vi "3.手柄操作发送指令至TCP服务器.vi"() -> ()   [LabVIEW 2018]
uses:
  <vilib>/Utility/inputDevices.llb/joystickAcquire.vi
panel:
  in  "摄像头云台复位":bool
  in  "运动控制复位":bool
  in  "摄像头云台负向1":bool
  in  "摄像头云台正向1":bool
  in  "摄像头正向2":bool
  in  "摄像头负向2":bool
  in  "机械手扩展":bool
  in  "机械手夹紧":bool
  in  "重新采样":bool
  in  "水下采样":bool
  in  "右旋":bool
  in  "左旋":bool
  in  "右翻":bool
  in  "左翻":bool
  in  "下潜":bool
  in  "上浮":bool
  in  "后退":bool
  in  "右移":bool
  in  "左移":bool
  in  "前进":bool
  out "接收字符串":string
  out "开始flag":bool=TRUE
  in  "?":string="8088"
  in  "?":string="192.168.1.30"
  # "地   址："
  # "端口号："
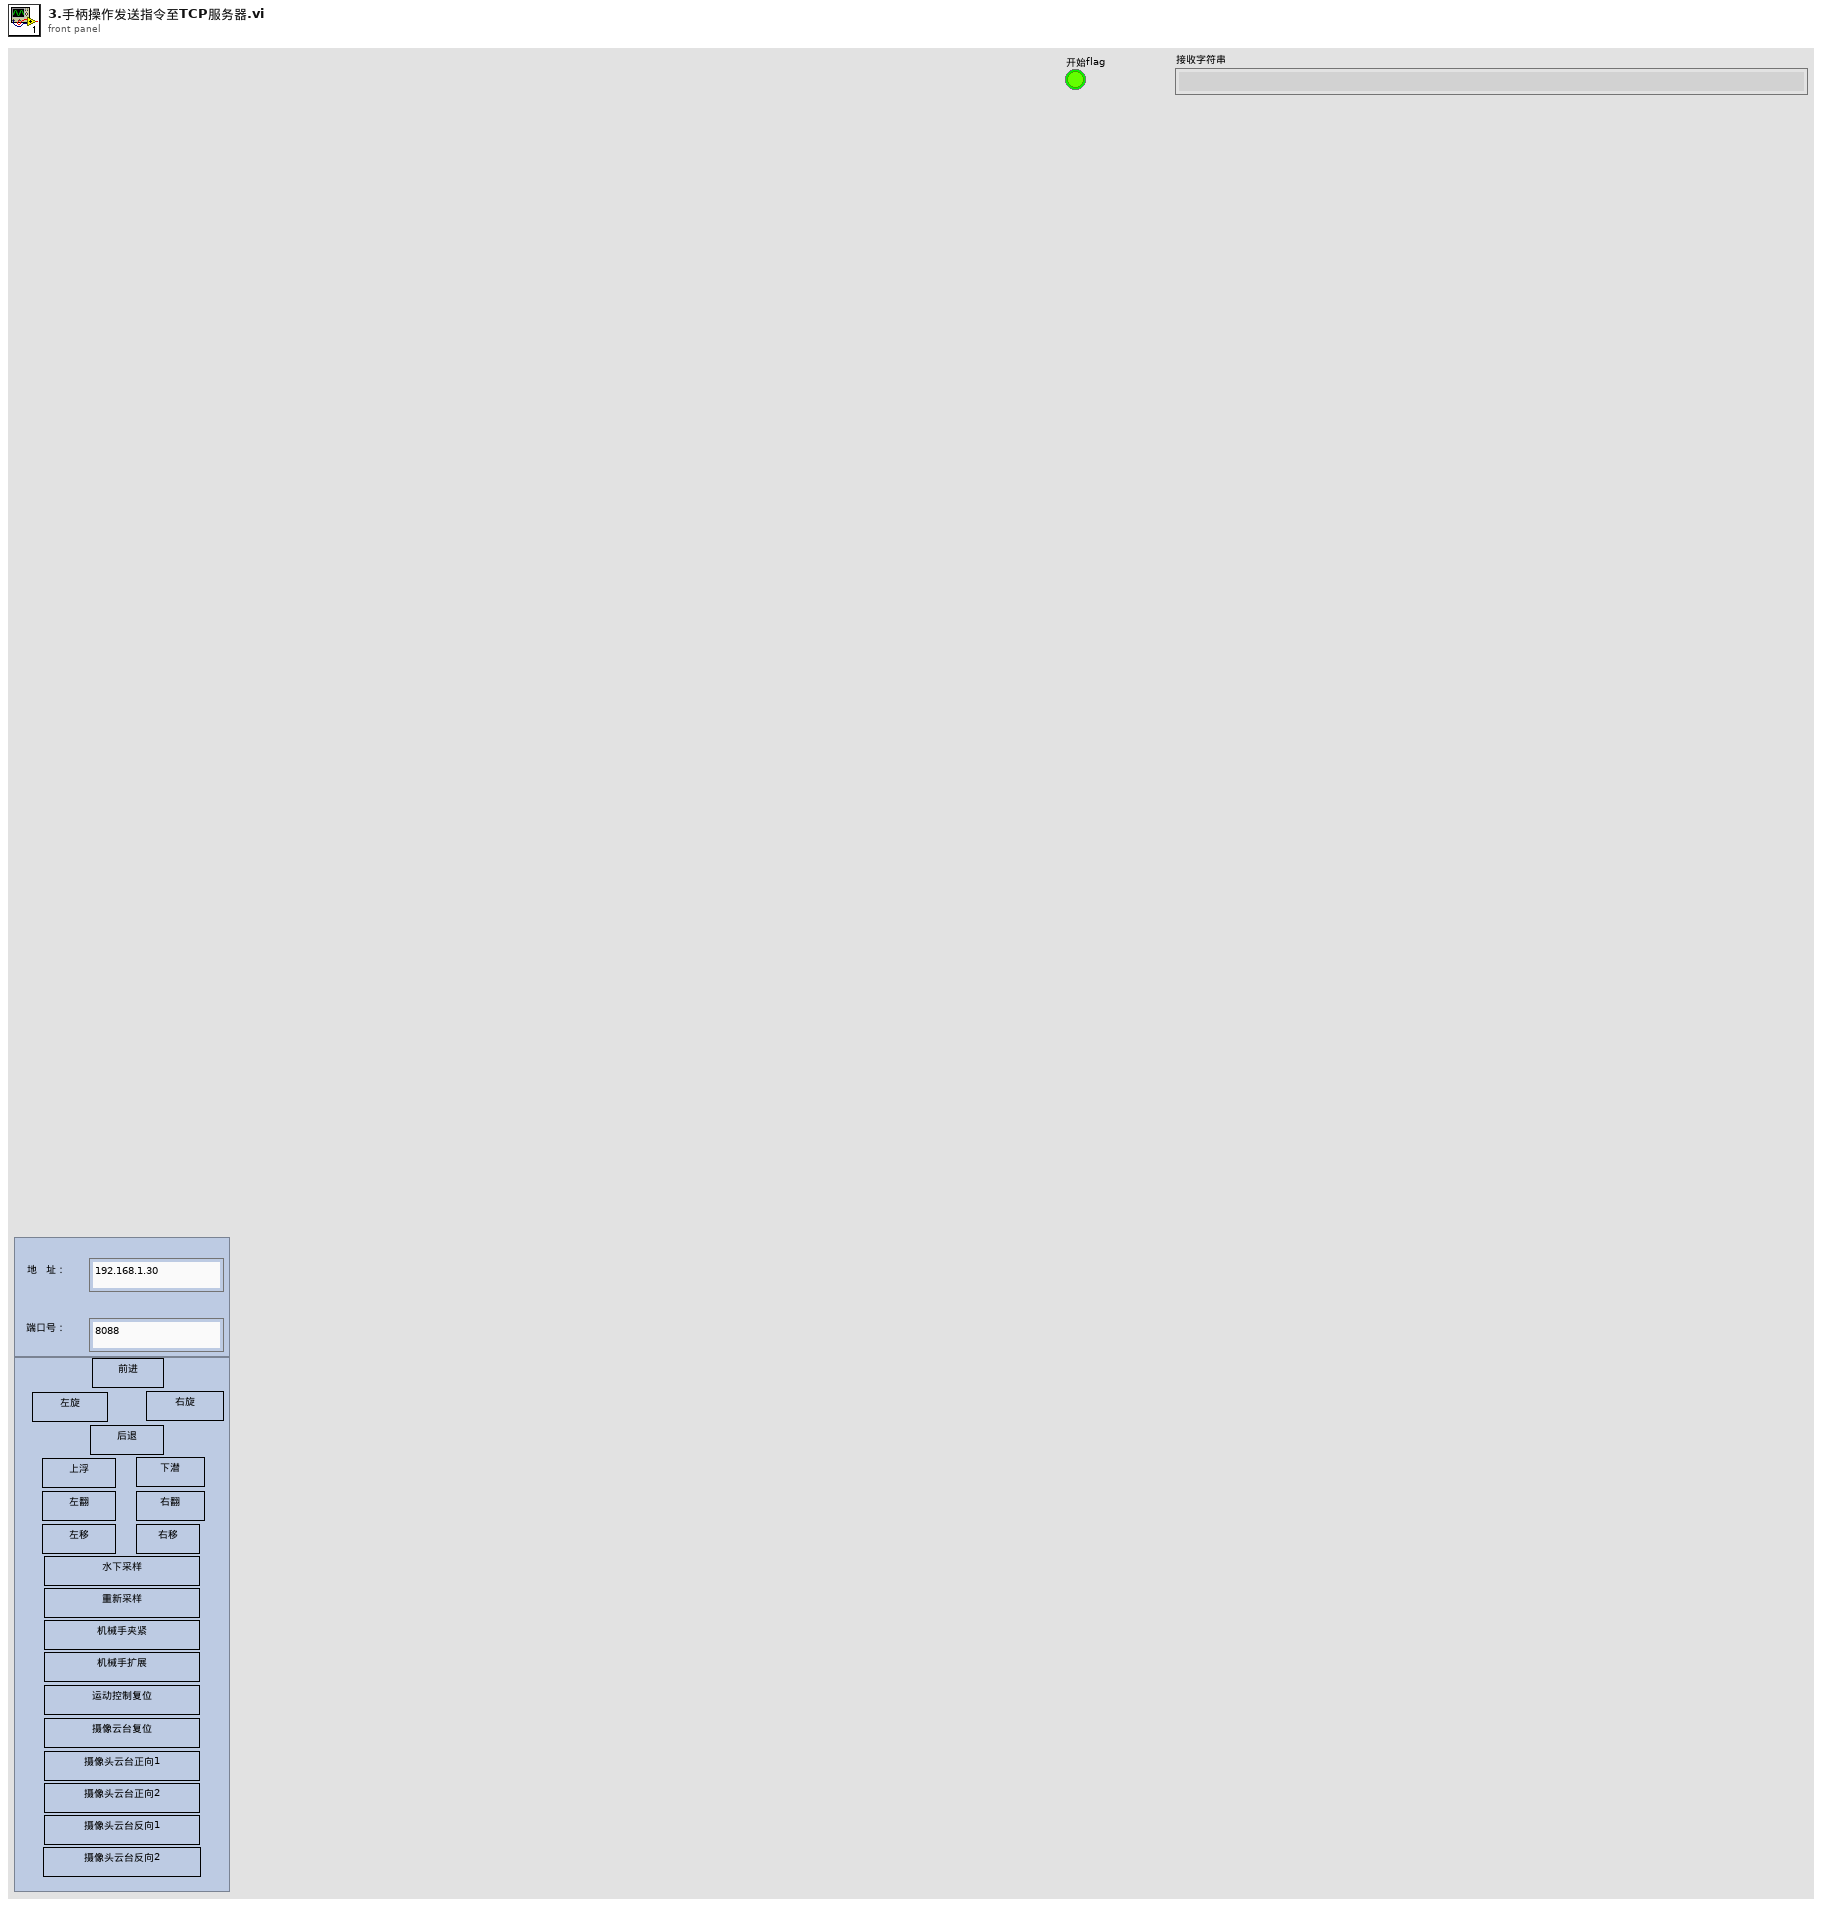
[diagram p1: front panel]
types:
  T1 = cluster{"X axis":i32, "Y axis":i32, "Z axis":i32, "X axis rotation":i32, "Y axis rotation":i32, "Z axis rotation":i32, "U axis":i32, "V axis":i32}
  T2 = cluster{"button 1":bool, "button 2":bool, "button 3":bool, "button 4":bool, "button 5":bool, "button 6":bool, "button 7":bool, "button 8":bool, "button 9":bool, "button 10":bool, "button 11":bool, "button 12":bool, "button 13":bool, "button 14":bool, "button 15":bool, "button 16":bool, "button 17":bool, "button 18":bool, "button 19":bool, "button 20":bool, "button 21":bool, "button 22":bool, "button 23":bool, "button 24":bool, "button 25":bool, "button 26":bool, "button 27":bool, "button 28":bool, "button 29":bool, "button 30":bool, "button 31":bool, "button 32":bool}
  T3 = cluster{"pov 1":i32, "pov 2":i32, "pov 3":i32, "pov 4":i32}
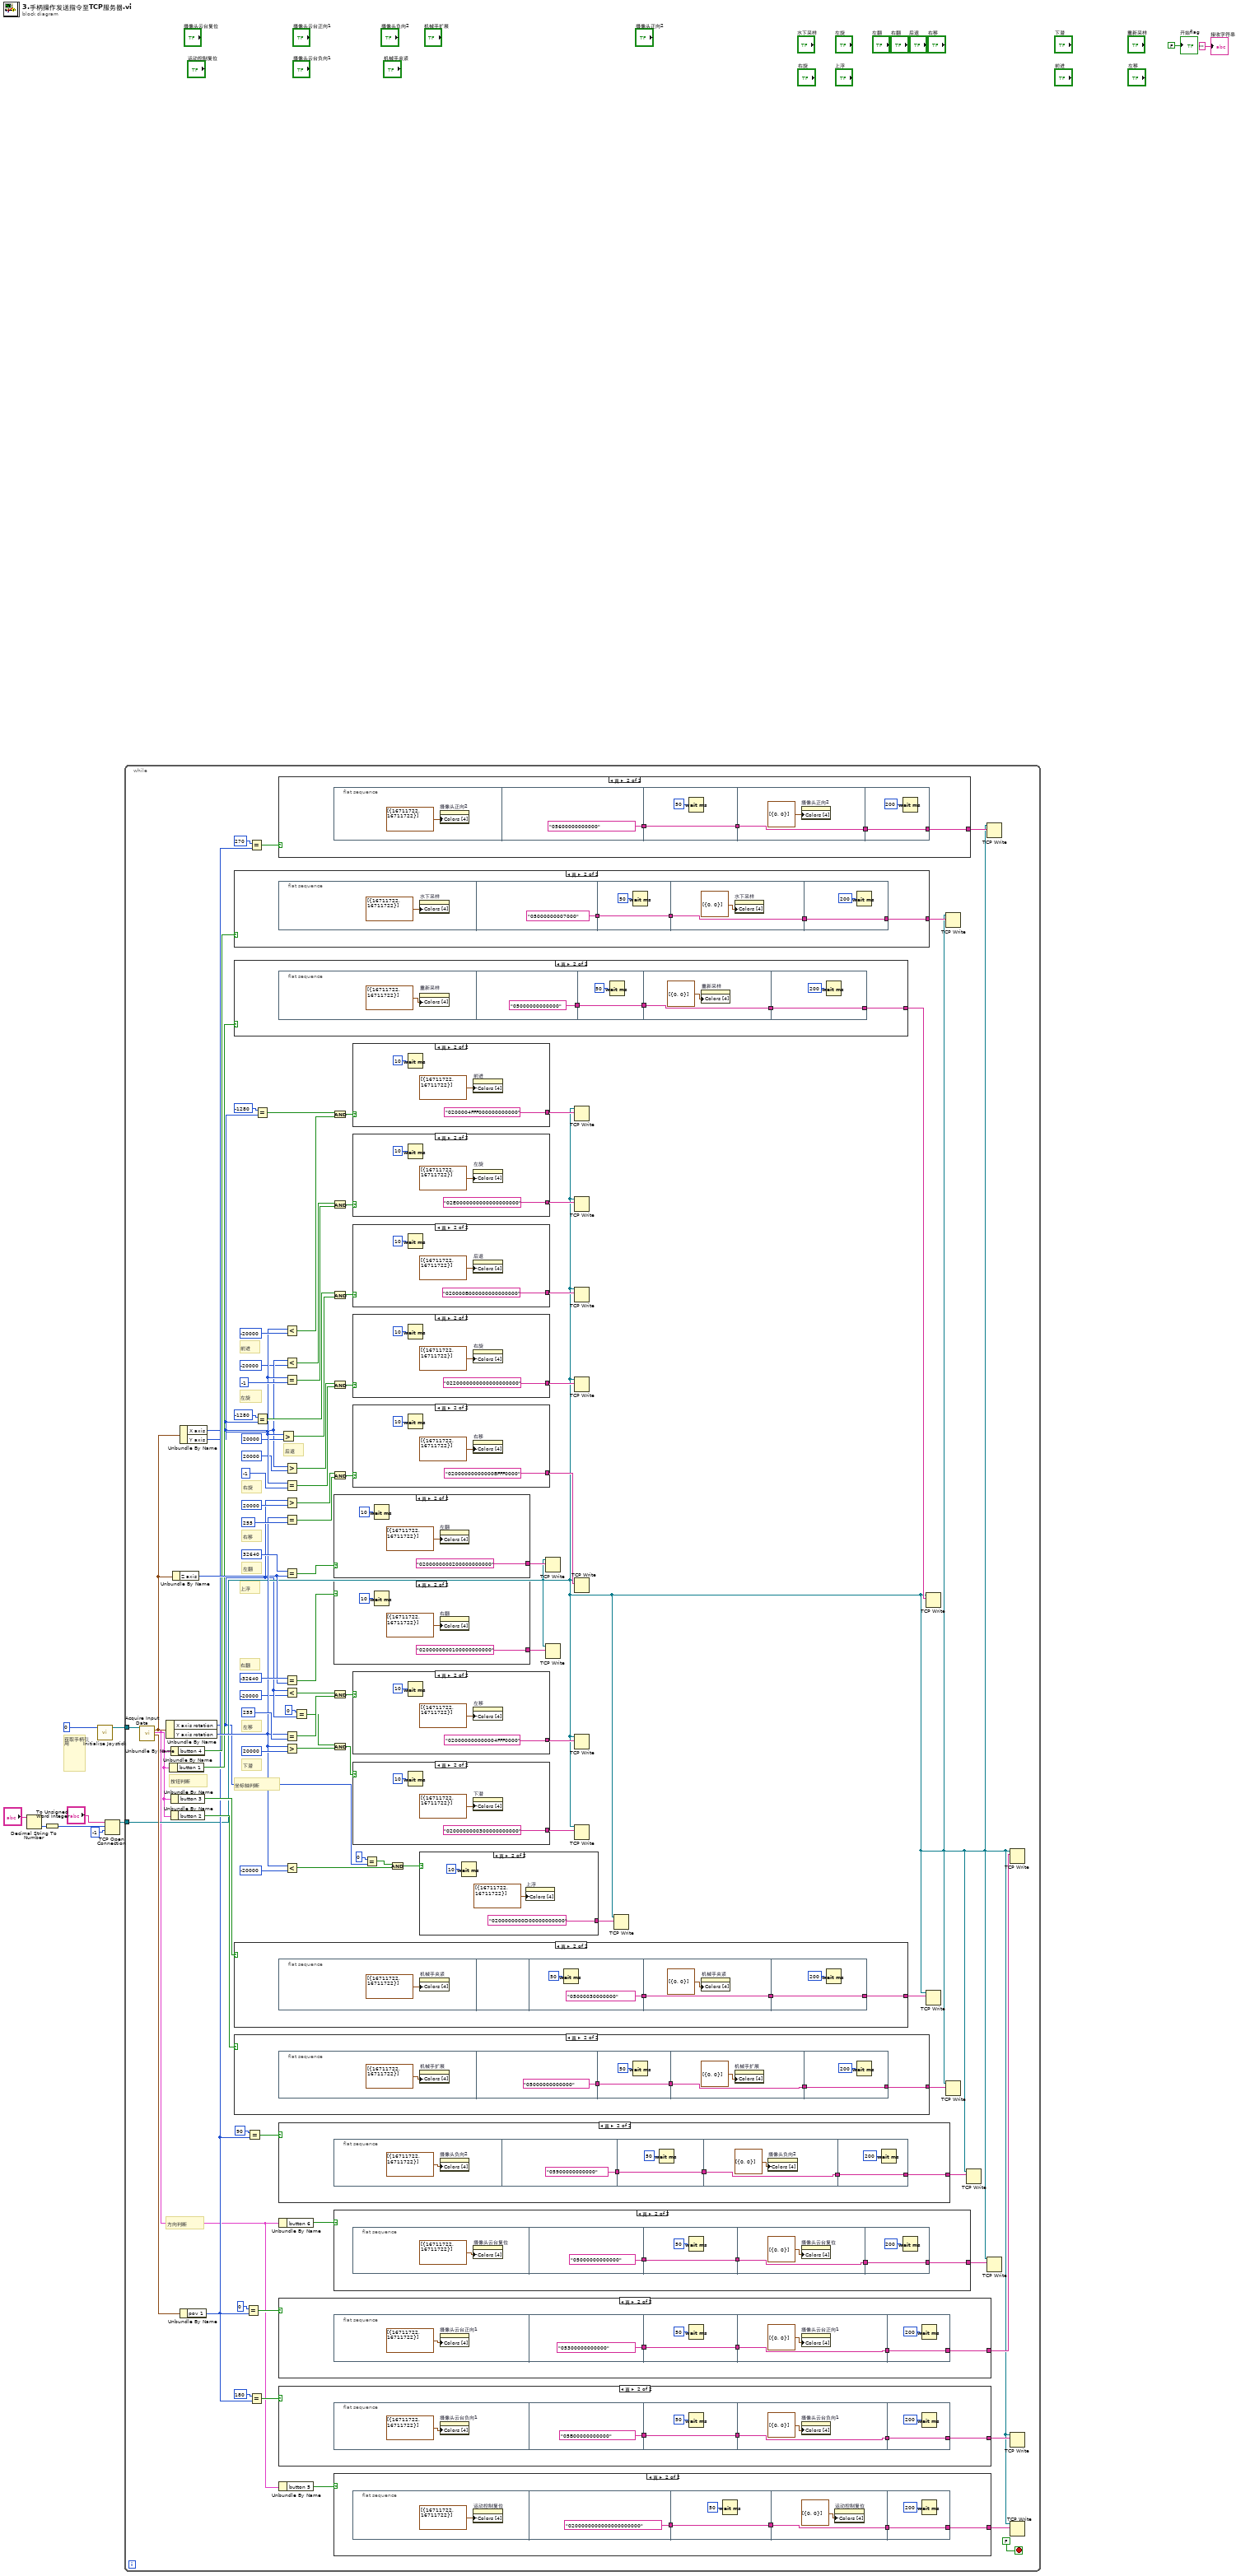
[diagram p0: block diagram]
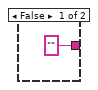
[diagram p2: hidden frame]
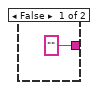
[diagram p3: hidden frame]
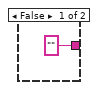
[diagram p4: hidden frame]
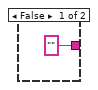
[diagram p5: hidden frame]
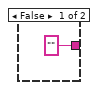
[diagram p6: hidden frame]
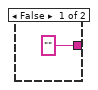
[diagram p7: hidden frame]
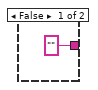
[diagram p8: hidden frame]
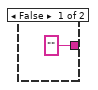
[diagram p9: hidden frame]
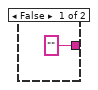
[diagram p10: hidden frame]
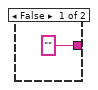
[diagram p11: hidden frame]
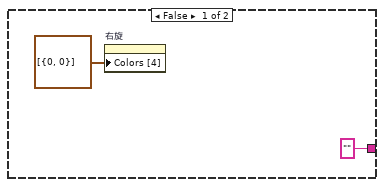
[diagram p12: hidden frame]
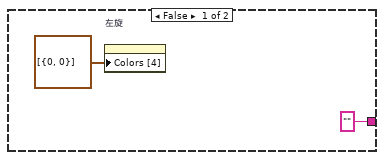
[diagram p13: hidden frame]
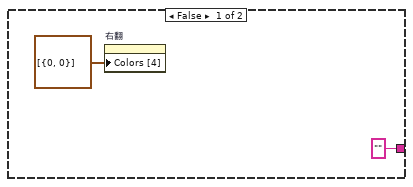
[diagram p14: hidden frame]
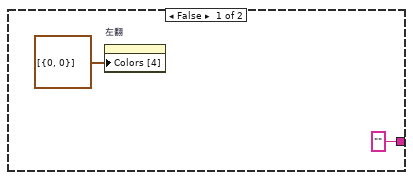
[diagram p15: hidden frame]
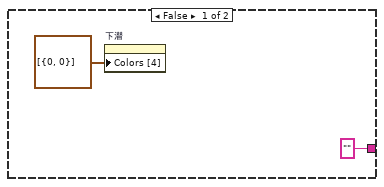
[diagram p16: hidden frame]
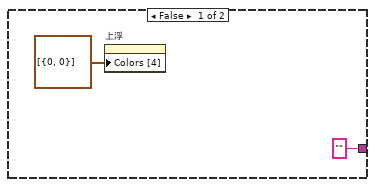
[diagram p17: hidden frame]
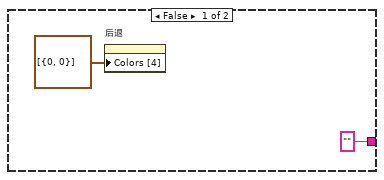
[diagram p18: hidden frame]
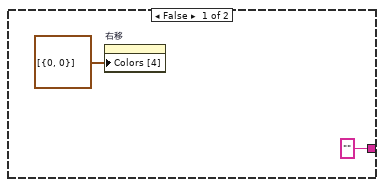
[diagram p19: hidden frame]
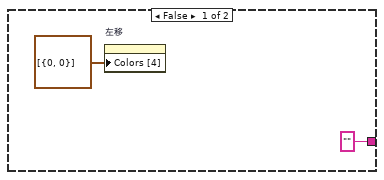
[diagram p20: hidden frame]
diagram:
  # "获取手柄引用"
  n1 = Decimal String To Number(string="?") -> (number=w6:i32)  [unwired: 2 in, 1 out]
  n2 = To Unsigned Word Integer(number=w6) -> (unsigned 16bit integer=w5:u16)
  n3 = call <vilib>:"Initialize Joystick.vi"("device index"=0) -> ("device ID"=w1:refnum<k1>)  [unwired: 9 in, 1 out]
  n4 = TCP Open Connection(address="?", remote port or service name=w5, timeout ms (60000)=-1 ("超时毫秒(60000)")) -> (connection ID=w4:refnum<k5>)  [unwired: 2 in, 1 out]
  n5 = while {
    tunnel: w4 -> [w31]
    tunnel: w1 -> [w12]
    stop <- FALSE stop-if-true
    # "方向判断"
    # "按钮判断"
    # "坐标轴判断"
    # "左翻"
    # "右旋"
    # "左旋"
    # "右翻"
    # "下潜"
    # "上浮"
    # "后退"
    # "右移"
    # "左移"
    # "前进"
    n6 = call-poly <vilib>:"Acquire Input Data.vi"("device ID"=w12) -> ("axis info"=w65:T1, "button info"=w13:T2, "direction info"=w60:T3)  [unwired: 14 in, 2 out]
    n7 = Unbundle By Name(w65) -> ("X axis rotation"=w15:i32, "Y axis rotation"=w69:i32)
    n8 = Unbundle By Name(w13) -> ("button 1"=w63:bool)
    n9 = Unbundle By Name(w13) -> ("button 4"=w64:bool)
    n10 = Unbundle By Name(w13) -> ("button 3"=w62:bool)
    n11 = Unbundle By Name(w13) -> ("button 2"=w61:bool)
    n12 = Unbundle By Name(w65) -> ("Z axis"=w66:i32)
    n13 = Unbundle By Name(w65) -> ("X axis"=w18:i32, "Y axis"=w23:i32)
    n14 = Unbundle By Name(w60) -> ("pov 1"=w56:i32)
    n15 = case shown="真" w64 {
      tunnel: ["" w217] -> w40
      frame False {
      }
      frame True {
        n16 = flat-sequence {
          tunnel: ["05000000007000"] -> w220
          tunnel: w220 -> [w223]
          tunnel: [w223] -> w219
          tunnel: w219 -> [w225]
          tunnel: [w225] -> w218
          tunnel: w218 -> [w227]
          tunnel: [w227] -> w217
          frame #0 {
            n17 = property on="水下采样" class="Bool"("Colors [4]"=cluster{u32, u32}[] [{16711722, 16711722}] ("颜色[4]")) -> ()  [unwired: 2 in, 2 out]
          }
          frame #1 {
          }
          frame #2 {
            n18 = Wait (ms)(milliseconds to wait=u32 50 ("等待时间（毫秒）")) -> ()  [unwired: 1 out]
          }
          frame #3 {
            n19 = property on="水下采样" class="Bool"("Colors [4]"=cluster{u32, u32}[] [{0, 0}] ("颜色[4]")) -> ()  [unwired: 2 in, 2 out]
          }
          frame #4 {
            n20 = Wait (ms)(milliseconds to wait=u32 200 ("等待时间（毫秒）")) -> ()  [unwired: 1 out]
          }
        }
      }
    }
    n21 = case shown="真" w63 {
      tunnel: ["" w193] -> w41
      frame False {
      }
      frame True {
        n22 = flat-sequence {
          tunnel: ["05000000000000"] -> w191
          tunnel: [w197] -> w194
          tunnel: w191 -> [w197]
          tunnel: w194 -> [w199]
          tunnel: [w199] -> w192
          tunnel: [w202] -> w193
          tunnel: w192 -> [w202]
          frame #0 {
            n23 = property on="重新采样" class="Bool"("Colors [4]"=cluster{u32, u32}[] [{16711722, 16711722}] ("颜色[4]")) -> ()  [unwired: 2 in, 2 out]
          }
          frame #1 {
          }
          frame #2 {
            n24 = Wait (ms)(milliseconds to wait=u32 50 ("等待时间（毫秒）")) -> ()  [unwired: 1 out]
          }
          frame #3 {
            n25 = property on="重新采样" class="Bool"("Colors [4]"=cluster{u32, u32}[] [{0, 0}] ("颜色[4]")) -> ()  [unwired: 2 in, 2 out]
          }
          frame #4 {
            n26 = Wait (ms)(milliseconds to wait=u32 200 ("等待时间（毫秒）")) -> ()  [unwired: 1 out]
          }
        }
      }
    }
    n27 = case shown="真" w62 {
      tunnel: ["" w180] -> w39
      frame False {
      }
      frame True {
        n28 = flat-sequence {
          tunnel: ["05000030000000"] -> w182
          tunnel: w182 -> [w186]
          tunnel: [w186] -> w181
          tunnel: w181 -> [w188]
          tunnel: [w188] -> w180
          frame #0 {
            n29 = property on="机械手夹紧" class="Bool"("Colors [4]"=cluster{u32, u32}[] [{16711722, 16711722}] ("颜色[4]")) -> ()  [unwired: 2 in, 2 out]
          }
          frame #1 {
          }
          frame #2 {
            n30 = Wait (ms)(milliseconds to wait=u32 50 ("等待时间（毫秒）")) -> ()  [unwired: 1 out]
          }
          frame #3 {
            n31 = property on="机械手夹紧" class="Bool"("Colors [4]"=cluster{u32, u32}[] [{0, 0}] ("颜色[4]")) -> ()  [unwired: 2 in, 2 out]
          }
          frame #4 {
            n32 = Wait (ms)(milliseconds to wait=u32 200 ("等待时间（毫秒）")) -> ()  [unwired: 1 out]
          }
        }
      }
    }
    n33 = case shown="真" w61 {
      tunnel: ["" w167] -> w38
      frame False {
      }
      frame True {
        n34 = flat-sequence {
          tunnel: ["05000000000000"] -> w170
          tunnel: w170 -> [w173]
          tunnel: [w173] -> w169
          tunnel: w169 -> [w175]
          tunnel: [w175] -> w168
          tunnel: w168 -> [w177]
          tunnel: [w177] -> w167
          frame #0 {
            n35 = property on="机械手扩展" class="Bool"("Colors [4]"=cluster{u32, u32}[] [{16711722, 16711722}] ("颜色[4]")) -> ()  [unwired: 2 in, 2 out]
          }
          frame #1 {
          }
          frame #2 {
            n36 = Wait (ms)(milliseconds to wait=u32 50 ("等待时间（毫秒）")) -> ()  [unwired: 1 out]
          }
          frame #3 {
            n37 = property on="机械手扩展" class="Bool"("Colors [4]"=cluster{u32, u32}[] [{0, 0}] ("颜色[4]")) -> ()  [unwired: 2 in, 2 out]
          }
          frame #4 {
            n38 = Wait (ms)(milliseconds to wait=u32 200 ("等待时间（毫秒）")) -> ()  [unwired: 1 out]
          }
        }
      }
    }
    n39 = Equal?(x=0, y=w56) -> (x = y?=w54:bool)
    n40 = Equal?(x=90, y=w56) -> (x = y?=w51:bool)
    n41 = Equal?(x=270, y=w56) -> (x = y?=w53:bool)
    n42 = Equal?(x=180, y=w56) -> (x = y?=w52:bool)
    n43 = Equal?(x=-1280, y=w18) -> (x = y?=w98:bool)
    n44 = Equal?(x=-1280, y=w18) -> (x = y?=w95:bool)
    n45 = case shown="真" w53 {
      tunnel: ["" w154] -> w36
      frame False {
      }
      frame True {
        n46 = flat-sequence {
          tunnel: ["05600000000000"] -> w157
          tunnel: w157 -> [w160]
          tunnel: [w160] -> w156
          tunnel: w156 -> [w162]
          tunnel: [w162] -> w155
          tunnel: w155 -> [w164]
          tunnel: [w164] -> w154
          frame #0 {
            n47 = property on="摄像头正向2" class="Bool"("Colors [4]"=cluster{u32, u32}[] [{16711722, 16711722}] ("颜色[4]")) -> ()  [unwired: 2 in, 2 out]
          }
          frame #1 {
          }
          frame #2 {
            n48 = Wait (ms)(milliseconds to wait=u32 50 ("等待时间（毫秒）")) -> ()  [unwired: 1 out]
          }
          frame #3 {
            n49 = property on="摄像头正向2" class="Bool"("Colors [4]"=cluster{u32, u32}[] [{0, 0}] ("颜色[4]")) -> ()  [unwired: 2 in, 2 out]
          }
          frame #4 {
            n50 = Wait (ms)(milliseconds to wait=u32 200 ("等待时间（毫秒）")) -> ()  [unwired: 1 out]
          }
        }
      }
    }
    n51 = case shown="真" w51 {
      tunnel: ["" w128] -> w34
      frame False {
      }
      frame True {
        n52 = flat-sequence {
          tunnel: ["05900000000000"] -> w131
          tunnel: w131 -> [w134]
          tunnel: [w134] -> w130
          tunnel: w130 -> [w136]
          tunnel: [w136] -> w129
          tunnel: w129 -> [w138]
          tunnel: [w138] -> w128
          frame #0 {
            n53 = property on="摄像头负向2" class="Bool"("Colors [4]"=cluster{u32, u32}[] [{16711722, 16711722}] ("颜色[4]")) -> ()  [unwired: 2 in, 2 out]
          }
          frame #1 {
          }
          frame #2 {
            n54 = Wait (ms)(milliseconds to wait=u32 50 ("等待时间（毫秒）")) -> ()  [unwired: 1 out]
          }
          frame #3 {
            n55 = property on="摄像头负向2" class="Bool"("Colors [4]"=cluster{u32, u32}[] [{0, 0}] ("颜色[4]")) -> ()  [unwired: 2 in, 2 out]
          }
          frame #4 {
            n56 = Wait (ms)(milliseconds to wait=u32 200 ("等待时间（毫秒）")) -> ()  [unwired: 1 out]
          }
        }
      }
    }
    n57 = Unbundle By Name(w13) -> ("button 6"=w29:bool)
    n58 = case shown="真" w54 {
      tunnel: ["" w204] -> w37
      frame False {
      }
      frame True {
        n59 = flat-sequence {
          tunnel: ["05300000000000"] -> w207
          tunnel: w207 -> [w210]
          tunnel: [w210] -> w206
          tunnel: w206 -> [w212]
          tunnel: [w212] -> w205
          tunnel: w205 -> [w214]
          tunnel: [w214] -> w204
          frame #0 {
            n60 = property on="摄像头云台正向1" class="Bool"("Colors [4]"=cluster{u32, u32}[] [{16711722, 16711722}] ("颜色[4]")) -> ()  [unwired: 2 in, 2 out]
          }
          frame #1 {
          }
          frame #2 {
            n61 = Wait (ms)(milliseconds to wait=u32 50 ("等待时间（毫秒）")) -> ()  [unwired: 1 out]
          }
          frame #3 {
            n62 = property on="摄像头云台正向1" class="Bool"("Colors [4]"=cluster{u32, u32}[] [{0, 0}] ("颜色[4]")) -> ()  [unwired: 2 in, 2 out]
          }
          frame #4 {
            n63 = Wait (ms)(milliseconds to wait=u32 200 ("等待时间（毫秒）")) -> ()  [unwired: 1 out]
          }
        }
      }
    }
    n64 = case shown="真" w52 {
      tunnel: ["" w141] -> w35
      frame False {
      }
      frame True {
        n65 = flat-sequence {
          tunnel: ["05B00000000000"] -> w144
          tunnel: w144 -> [w147]
          tunnel: [w147] -> w143
          tunnel: w143 -> [w149]
          tunnel: [w149] -> w142
          tunnel: w142 -> [w151]
          tunnel: [w151] -> w141
          frame #0 {
            n66 = property on="摄像头云台负向1" class="Bool"("Colors [4]"=cluster{u32, u32}[] [{16711722, 16711722}] ("颜色[4]")) -> ()  [unwired: 2 in, 2 out]
          }
          frame #1 {
          }
          frame #2 {
            n67 = Wait (ms)(milliseconds to wait=u32 50 ("等待时间（毫秒）")) -> ()  [unwired: 1 out]
          }
          frame #3 {
            n68 = property on="摄像头云台负向1" class="Bool"("Colors [4]"=cluster{u32, u32}[] [{0, 0}] ("颜色[4]")) -> ()  [unwired: 2 in, 2 out]
          }
          frame #4 {
            n69 = Wait (ms)(milliseconds to wait=u32 200 ("等待时间（毫秒）")) -> ()  [unwired: 1 out]
          }
        }
      }
    }
    n70 = Unbundle By Name(w13) -> ("button 5"=w30:bool)
    n71 = Greater?(x=w23, y=20000) -> (0:w24:bool)
    n72 = Less?(x=w23, y=-20000) -> (x < y?=w26:bool)
    n73 = Less?(x=w18, y=-20000 ("x")) -> (x < y?=w19:bool)
    n74 = Equal?(x=w23, y=-1) -> (x = y?=w93:bool)
    n75 = Greater?(x=w18, y=20000 ("x")) -> (0:w20:bool)
    n76 = Equal?(x=w23, y=-1) -> (x = y?=w91:bool)
    n77 = Greater?(x=w15, y=20000 ("x")) -> (0:w83:bool)
    n78 = Equal?(x=w69, y=255) -> (x = y?=w84:bool)
    n79 = Equal?(x=32640, y=w66) -> (x = y?=w68:bool)
    n80 = Equal?(x=-32640, y=w66) -> (x = y?=w67:bool)
    n81 = Less?(x=w15, y=-20000 ("x")) -> (x < y?=w86:bool)
    n82 = Equal?(x=w69, y=255) -> (x = y?=w87:bool)
    n83 = Greater?(x=w69, y=20000) -> (0:w71:bool)
    n84 = Less?(x=w69, y=-20000) -> (x < y?=w76:bool)
    n85 = Equal?(x=0, y=w15) -> (x = y?=w70:bool)
    n86 = And(x=w98, y=w26) -> (x .and. y?=w97:bool)
    n87 = And(x=w19, y=w93) -> (x .and. y?=w33:bool)
    n88 = And(x=w95, y=w24) -> (x .and. y?=w90:bool)
    n89 = And(x=w20, y=w91) -> (x .and. y?=w89:bool)
    n90 = And(x=w83, y=w84) -> (x .and. y?=w79:bool)
    n91 = And(x=w86, y=w87) -> (x .and. y?=w80:bool)
    n92 = And(x=w70, y=w71) -> (x .and. y?=w32:bool)
    n93 = case shown="真" w68 {
      tunnel: ["" "0200000000200000000000"] -> w43
      frame False {
        n94 = property on="左翻" class="Bool"("Colors [4]"=cluster{u32, u32}[] [{0, 0}] ("颜色[4]")) -> ()  [unwired: 2 in, 2 out]
      }
      frame True {
        n95 = Wait (ms)(milliseconds to wait=u32 10 ("等待时间（毫秒）")) -> ()  [unwired: 1 out]
        n96 = property on="左翻" class="Bool"("Colors [4]"=cluster{u32, u32}[] [{16711722, 16711722}] ("颜色[4]")) -> ()  [unwired: 2 in, 2 out]
      }
    }
    n97 = case shown="真" w67 {
      tunnel: ["" "0200000000100000000000"] -> w42
      frame False {
        n98 = property on="右翻" class="Bool"("Colors [4]"=cluster{u32, u32}[] [{0, 0}] ("颜色[4]")) -> ()  [unwired: 2 in, 2 out]
      }
      frame True {
        n99 = Wait (ms)(milliseconds to wait=u32 10 ("等待时间（毫秒）")) -> ()  [unwired: 1 out]
        n100 = property on="右翻" class="Bool"("Colors [4]"=cluster{u32, u32}[] [{16711722, 16711722}] ("颜色[4]")) -> ()  [unwired: 2 in, 2 out]
      }
    }
    n101 = case shown="真" w29 {
      tunnel: ["" w102] -> w28
      frame False {
      }
      frame True {
        n102 = flat-sequence {
          tunnel: ["05000000000000"] -> w105
          tunnel: w105 -> [w108]
          tunnel: [w108] -> w104
          tunnel: w104 -> [w110]
          tunnel: [w110] -> w103
          tunnel: w103 -> [w112]
          tunnel: [w112] -> w102
          frame #0 {
            n103 = property on="摄像头云台复位" class="Bool"("Colors [4]"=cluster{u32, u32}[] [{16711722, 16711722}] ("颜色[4]")) -> ()  [unwired: 2 in, 2 out]
          }
          frame #1 {
          }
          frame #2 {
            n104 = Wait (ms)(milliseconds to wait=u32 50 ("等待时间（毫秒）")) -> ()  [unwired: 1 out]
          }
          frame #3 {
            n105 = property on="摄像头云台复位" class="Bool"("Colors [4]"=cluster{u32, u32}[] [{0, 0}] ("颜色[4]")) -> ()  [unwired: 2 in, 2 out]
          }
          frame #4 {
            n106 = Wait (ms)(milliseconds to wait=u32 200 ("等待时间（毫秒）")) -> ()  [unwired: 1 out]
          }
        }
      }
    }
    n107 = case shown="真" w30 {
      tunnel: ["" w115] -> w27
      frame False {
      }
      frame True {
        n108 = flat-sequence {
          tunnel: ["0200000000000000000000"] -> w118
          tunnel: w118 -> [w121]
          tunnel: [w121] -> w117
          tunnel: w117 -> [w123]
          tunnel: [w123] -> w116
          tunnel: w116 -> [w125]
          tunnel: [w125] -> w115
          frame #0 {
            n109 = property on="运动控制复位" class="Bool"("Colors [4]"=cluster{u32, u32}[] [{16711722, 16711722}] ("颜色[4]")) -> ()  [unwired: 2 in, 2 out]
          }
          frame #1 {
          }
          frame #2 {
            n110 = Wait (ms)(milliseconds to wait=u32 50 ("等待时间（毫秒）")) -> ()  [unwired: 1 out]
          }
          frame #3 {
            n111 = property on="运动控制复位" class="Bool"("Colors [4]"=cluster{u32, u32}[] [{0, 0}] ("颜色[4]")) -> ()  [unwired: 2 in, 2 out]
          }
          frame #4 {
            n112 = Wait (ms)(milliseconds to wait=u32 200 ("等待时间（毫秒）")) -> ()  [unwired: 1 out]
          }
        }
      }
    }
    n113 = case shown="真" w97 {
      tunnel: ["" "0200004FFF000000000000"] -> w50
      frame False {
        n114 = property on="前进" class="Bool"("Colors [4]"=cluster{u32, u32}[] [{0, 0}] ("颜色[4]")) -> ()  [unwired: 2 in, 2 out]
      }
      frame True {
        n115 = Wait (ms)(milliseconds to wait=u32 10 ("等待时间（毫秒）")) -> ()  [unwired: 1 out]
        n116 = property on="前进" class="Bool"("Colors [4]"=cluster{u32, u32}[] [{16711722, 16711722}] ("颜色[4]")) -> ()  [unwired: 2 in, 2 out]
      }
    }
    n117 = case shown="真" w33 {
      tunnel: ["" "02E0000000000000000000"] -> w48
      frame False {
        n118 = property on="左旋" class="Bool"("Colors [4]"=cluster{u32, u32}[] [{0, 0}] ("颜色[4]")) -> ()  [unwired: 2 in, 2 out]
      }
      frame True {
        n119 = Wait (ms)(milliseconds to wait=u32 10 ("等待时间（毫秒）")) -> ()  [unwired: 1 out]
        n120 = property on="左旋" class="Bool"("Colors [4]"=cluster{u32, u32}[] [{16711722, 16711722}] ("颜色[4]")) -> ()  [unwired: 2 in, 2 out]
      }
    }
    n121 = case shown="真" w90 {
      tunnel: ["" "020000B000000000000000"] -> w49
      frame False {
        n122 = property on="后退" class="Bool"("Colors [4]"=cluster{u32, u32}[] [{0, 0}] ("颜色[4]")) -> ()  [unwired: 2 in, 2 out]
      }
      frame True {
        n123 = Wait (ms)(milliseconds to wait=u32 10 ("等待时间（毫秒）")) -> ()  [unwired: 1 out]
        n124 = property on="后退" class="Bool"("Colors [4]"=cluster{u32, u32}[] [{16711722, 16711722}] ("颜色[4]")) -> ()  [unwired: 2 in, 2 out]
      }
    }
    n125 = case shown="真" w89 {
      tunnel: ["" "0220000000000000000000"] -> w47
      frame False {
        n126 = property on="右旋" class="Bool"("Colors [4]"=cluster{u32, u32}[] [{0, 0}] ("颜色[4]")) -> ()  [unwired: 2 in, 2 out]
      }
      frame True {
        n127 = Wait (ms)(milliseconds to wait=u32 10 ("等待时间（毫秒）")) -> ()  [unwired: 1 out]
        n128 = property on="右旋" class="Bool"("Colors [4]"=cluster{u32, u32}[] [{16711722, 16711722}] ("颜色[4]")) -> ()  [unwired: 2 in, 2 out]
      }
    }
    n129 = case shown="真" w79 {
      tunnel: ["" "02000000000000BFFF0000"] -> w45
      frame False {
        n130 = property on="右移" class="Bool"("Colors [4]"=cluster{u32, u32}[] [{0, 0}] ("颜色[4]")) -> ()  [unwired: 2 in, 2 out]
      }
      frame True {
        n131 = Wait (ms)(milliseconds to wait=u32 10 ("等待时间（毫秒）")) -> ()  [unwired: 1 out]
        n132 = property on="右移" class="Bool"("Colors [4]"=cluster{u32, u32}[] [{16711722, 16711722}] ("颜色[4]")) -> ()  [unwired: 2 in, 2 out]
      }
    }
    n133 = case shown="真" w80 {
      tunnel: ["" "020000000000004FFF0000"] -> w46
      frame False {
        n134 = property on="左移" class="Bool"("Colors [4]"=cluster{u32, u32}[] [{0, 0}] ("颜色[4]")) -> ()  [unwired: 2 in, 2 out]
      }
      frame True {
        n135 = Wait (ms)(milliseconds to wait=u32 10 ("等待时间（毫秒）")) -> ()  [unwired: 1 out]
        n136 = property on="左移" class="Bool"("Colors [4]"=cluster{u32, u32}[] [{16711722, 16711722}] ("颜色[4]")) -> ()  [unwired: 2 in, 2 out]
      }
    }
    n137 = case shown="真" w32 {
      tunnel: ["" "0200000000300000000000"] -> w11
      frame False {
        n138 = property on="下潜" class="Bool"("Colors [4]"=cluster{u32, u32}[] [{0, 0}] ("颜色[4]")) -> ()  [unwired: 2 in, 2 out]
      }
      frame True {
        n139 = Wait (ms)(milliseconds to wait=u32 10 ("等待时间（毫秒）")) -> ()  [unwired: 1 out]
        n140 = property on="下潜" class="Bool"("Colors [4]"=cluster{u32, u32}[] [{16711722, 16711722}] ("颜色[4]")) -> ()  [unwired: 2 in, 2 out]
      }
    }
    n141 = Equal?(x=0, y=w15) -> (x = y?=w75:bool)
    n142 = And(x=w75, y=w76) -> (x .and. y?=w74:bool)
    n143 = case shown="真" w74 {
      tunnel: ["" "0200000000D00000000000"] -> w44
      frame False {
        n144 = property on="上浮" class="Bool"("Colors [4]"=cluster{u32, u32}[] [{0, 0}] ("颜色[4]")) -> ()  [unwired: 2 in, 2 out]
      }
      frame True {
        n145 = Wait (ms)(milliseconds to wait=u32 10 ("等待时间（毫秒）")) -> ()  [unwired: 1 out]
        n146 = property on="上浮" class="Bool"("Colors [4]"=cluster{u32, u32}[] [{16711722, 16711722}] ("颜色[4]")) -> ()  [unwired: 2 in, 2 out]
      }
    }
    n147 = TCP Write(connection ID=w31, data in=w43) -> ()  [unwired: 2 in, 3 out]
    n148 = TCP Write(connection ID=w31, data in=w42) -> ()  [unwired: 2 in, 3 out]
    n149 = TCP Write(connection ID=w31, data in=w50) -> ()  [unwired: 2 in, 3 out]
    n150 = TCP Write(connection ID=w31, data in=w48) -> ()  [unwired: 2 in, 3 out]
    n151 = TCP Write(connection ID=w31, data in=w49) -> ()  [unwired: 2 in, 3 out]
    n152 = TCP Write(connection ID=w31, data in=w47) -> ()  [unwired: 2 in, 3 out]
    n153 = TCP Write(connection ID=w31, data in=w45) -> ()  [unwired: 2 in, 3 out]
    n154 = TCP Write(connection ID=w31, data in=w46) -> ()  [unwired: 2 in, 3 out]
    n155 = TCP Write(connection ID=w31, data in=w11) -> ()  [unwired: 2 in, 3 out]
    n156 = TCP Write(connection ID=w31, data in=w44) -> ()  [unwired: 2 in, 3 out]
    n157 = TCP Write(connection ID=w31, data in=w41) -> ()  [unwired: 2 in, 3 out]
    n158 = TCP Write(connection ID=w31, data in=w39) -> ()  [unwired: 2 in, 3 out]
    n159 = TCP Write(connection ID=w31, data in=w40) -> ()  [unwired: 2 in, 3 out]
    n160 = TCP Write(connection ID=w31, data in=w38) -> ()  [unwired: 2 in, 3 out]
    n161 = TCP Write(connection ID=w31, data in=w34) -> ()  [unwired: 2 in, 3 out]
    n162 = TCP Write(connection ID=w31, data in=w36) -> ()  [unwired: 2 in, 3 out]
    n163 = TCP Write(connection ID=w31, data in=w28) -> ()  [unwired: 2 in, 3 out]
    n164 = TCP Write(connection ID=w31, data in=w37) -> ()  [unwired: 2 in, 3 out]
    n165 = TCP Write(connection ID=w31, data in=w35) -> ()  [unwired: 2 in, 3 out]
    n166 = TCP Write(connection ID=w31, data in=w27) -> ()  [unwired: 2 in, 3 out]
  }
  "开始flag" <- FALSE ("布尔")
  "接收字符串" <- ""
